vi "Capacitance PID-LS370.vi"() -> ()   [LabVIEW 2020]
doc: "This VI is meant to be used with the process control package (PID controller) and an MIO-series or Lab-PC data acquisition board. Connect the analog output to the analog input through the resistor-capacitor network shown on the front panel (scroll down to view it). The VI attempts to adjust the analog output so that the input (process variable or PV) equals the setpoint (SP). SP and PV are displayed on a strip chart. You can experiment with different controller tuning methods and try for the fastest settling time with the least overshoot.\n\nThe input span is -10 to +10 V, or 20V = 100%. The output span is 0 to +10 V, or 10V = 100%. PV and SP are in Volts. Your MIO board should be set up for differential input and -10 to +10 V range; the output should be unipolar, 10V (these are all factory defaults). If you elect to use other settings, run the configuration VIs as necessary.\n\nThe recommended network has a DC gain of 0.33, an effective deadtime of about 5 Sec., and an effective time constant of about 30 Sec."
uses:
  <vilib>/addons/control/pid/NI_PID__autopid compat.lvlib
panel:
  out "Trend 2":dbl(graph)
  in  "Heater Range":i32(ring)=4 items=["Off", "31.6 uA", "100 uA", "316 uA", "1.00 mA", "3.16 mA", "10.0 mA", "31.6 mA", "100 mA"]
  in  "Heater Resistance(½)":dbl=400.0
  in  "Lakeshore GPIB Address":refnum<visa-resource-name>="GPIB0::12::INSTR"
  out "Cycle #":i32
  in  "Bias":dbl format="%.2f"
  in  "gain scheduling":T1={"gain schedule"=[40.0, 70.0, 100.0], "PID parameters"=[{"Kc"=20.0, "Ti (min)"=0.008, "Td (min)"=0.006}, {"Kc"=20.0, "Ti (min)"=0.008, "Td (min)"=0.006}, {"Kc"=20.0, "Ti (min)"=0.008, "Td (min)"=0.006}], "scheduling input"=0} {"scheduling input" items=["Setpoint", "Process variable", "Controller output", "Gain scheduling input"]; "PID parameters"."Td (min)" format="%.4f"; "PID parameters"."Ti (min)" format="%.4f"; "PID parameters"."Kc" format="%#.3f"; "gain schedule" format="%.2f"}
  in  "?":bool
  in  "options":T2={"sp low"=-10.0, "sp high"=10.0, "out low"=0.0, "out high"=10.0, "hold (F)"=FALSE, "auto (T)"=TRUE, "pro. band (F)"=FALSE, "reverse acting (T)"=TRUE, "beta"=1.0, "linearity"=1.0, "dt (s)"=-1.0} {"dt (s)" format="%.2f"; "linearity" min=0.0 max=1.0 format="%.2f"; "sp low" format="%.2f"; "sp high" format="%.2f"; "out low" format="%.2e"; "out high" format="%.2e"; "beta" min=0.0 max=1.0 format="%.2f"}
  in  "STOP":bool
  in  "Setpoint (pF)":dbl(slide)=3300.0 min=3350.0 max=3380.0 step=0.0001 scale=3350.0..3380.0 scale format="%.2f"
  out "Output (W)":dbl(slide) scale=0.0..0.025 scale format="%#.2p"
  in  "Cycle Time (sec)":dbl=0.5 format="%.2f"
  in  "Manual Out (W)":dbl(knob) min=-4e-06 max=4e-06 scale=-100.0..100.0 scale format="%#.2p"
  out "Trend":cluster{"Setpoint (V)":dbl, "Setpoint (V)":dbl}(graph)
  # "SP & PV range:"
  # "Output range:"
  # "-1: default,using\nsystem clock"
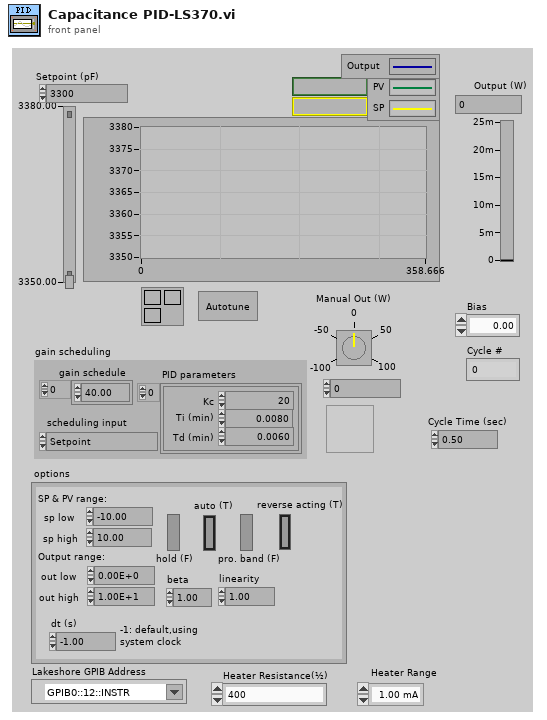
[diagram p1: front panel]
types:
  T1 = cluster{"gain schedule":dbl[], "PID parameters":cluster{"Kc":dbl, "Ti (min)":dbl, "Td (min)":dbl}[], "scheduling input":u16}
  T2 = cluster{"sp low":dbl, "sp high":dbl, "out low":dbl, "out high":dbl, "hold (F)":bool, "auto (T)":bool, "pro. band (F)":bool, "reverse acting (T)":bool, "beta":dbl, "linearity":dbl, "dt (s)":dbl}
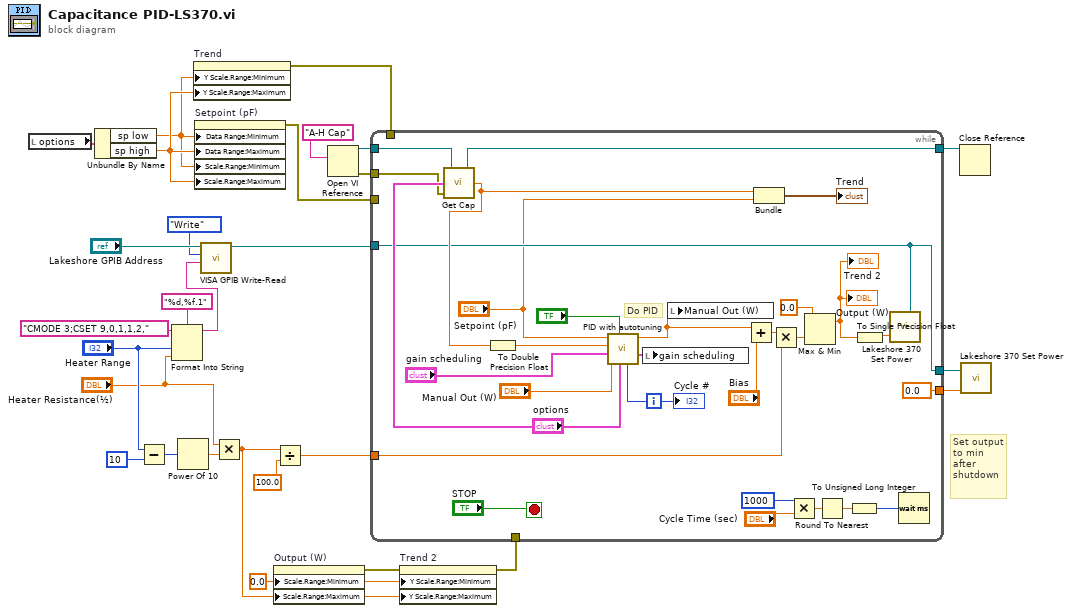
[diagram p0: block diagram]
diagram:
  w7 = 0.0 ("Scale.Range:Minimum")
  # "Set output \nto min after shutdown"
  n1 = local read "options"() -> (w11:T2)
  n2 = Unbundle By Name(w11) -> ("sp low"=w5:dbl, "sp high"=w6:dbl)
  n3 = Subtract(x="Heater Range", y=10) -> (x-y=w16:i32)
  n4 = Format Into String(format string="%d,%f.1" ("initial string"), initial string="CMODE 3;CSET 9,0,1,1,2,", "Heater Range", "Heater Resistance(½)") -> (resulting string=w18:string)  [unwired: 1 in, 1 out]
  n5 = Power Of 10(x=w16) -> (10^x=w13:dbl)
  n6 = property on="Trend" class="WFChart (strict)"("Y Scale.Range:Minimum"=w5, "Y Scale.Range:Maximum"=w6) -> (error out=w4:errorcluster)  [unwired: 2 in, 1 out]
  n7 = property on="Setpoint (pF)" class="Slide (strict)"("Data Range:Minimum"=w5, "Data Range:Maximum"=w6, "Scale.Range:Minimum"=w5, "Scale.Range:Maximum"=w6) -> (error out=w10:errorcluster)  [unwired: 2 in, 1 out]
  n8 = call "VISA GPIB Write-Read.vi"("Command"=w18, "Action"=enum16{"Write", "Read", "Write & Read"}."Write", "VISA resource name"="Lakeshore GPIB Address") -> ("dup VISA Session"=w21:refnum<visa-resource-name>)  [unwired: 5 in, 3 out]
  n9 = Multiply(x="Heater Resistance(½)", y=w13) -> (x*y=w3:dbl)
  n10 = property on="Output (W)" class="Slide (strict)"("Scale.Range:Minimum"=w7, "Scale.Range:Maximum"=w3) -> (error out=w9:errorcluster)  [unwired: 2 in, 1 out]
  n11 = Divide(x=w3, y=100.0) -> (x/y=w1:dbl)
  n12 = Open VI Reference(vi path="A-H Cap") -> (vi reference=w25:refnum<vi>, error out=w23:errorcluster)  [unwired: 5 in]
  n13 = property on="Trend 2" class="WFChart (strict)"(error in=w9, "Y Scale.Range:Minimum"=w7, "Y Scale.Range:Maximum"=w3) -> (error out=w8:errorcluster)  [unwired: 1 in, 1 out]
  n14 = while {
    tunnel: w23 -> [w43]
    tunnel: [w45] -> w24
    tunnel: w25 -> [w46]
    tunnel: [sgl 0.0] -> w27
    tunnel: [w36] -> w28
    tunnel: w21 -> [w36]
    tunnel: w10 -> [_]
    tunnel: w8 -> [_]
    tunnel: w4 -> [_]
    tunnel: w1 -> [w32]
    i -> [w51]
    stop <- "STOP" stop-if-true
    # "Do PID"
    n15 = call "Get Cap.vi"("error in"=w43, "options"="options", "VI Refnum 2"=w46) -> ("Setpoint (V)"=w42:dbl, "VI Refnum"=w45:refnum<vi>)  [unwired: 1 in]
    n16 = To Double Precision Float(number=w42) -> (double precision float=w47:dbl)
    n17 = call <vilib>:"PID with autotuning.vi"("iteration"=w51, "options"="options", "autotune? (F)"="?", "manual control"="Manual Out (W)", "gain scheduling"="gain scheduling", "process variable"=w47, "setpoint"="Setpoint (pF)") -> ("updated parameters"=w50:T1, "output"=w40:dbl)  [unwired: 2 in, 1 out]
    n18 = local write "gain scheduling"(w50) -> ()
    n19 = local write "Manual Out (W)"(w40) -> ()
    n20 = Add(x=w40, y="Bias") -> (x+y=w34:dbl)
    n21 = Bundle("Setpoint (V)"=w42, "Setpoint (pF)"="Setpoint (pF)") -> (→"Trend":cluster{"Setpoint (V)":dbl, "Setpoint (pF)":dbl})  [unwired: 1 in]
    n22 = Multiply(x=w34, y=w32) -> (x*y=w33:dbl)
    n23 = Multiply(x=1000, y="Cycle Time (sec)") -> (x*y=w54:dbl)
    n24 = Max & Min(x=0.0, y=w33) -> (max(x,y)=w30:dbl)  [unwired: 1 out]
    "Output (W)" <- w30
    "Trend 2" <- w30
    n25 = Round To Nearest(number=w54) -> (nearest integer value=w39:dbl)
    n26 = To Unsigned Long Integer(number=w39) -> (unsigned 32bit integer=w38:u32)
    n27 = To Single Precision Float(number=w30) -> (single precision float=w31:sgl)
    n28 = call "Lakeshore 370 Set Power.vi"("Heater Power (W)"=w31, "Lakeshore GPIB Address"=w36) -> ()
    n29 = Wait (ms)(milliseconds to wait=w38) -> ()  [unwired: 1 out]
    "Cycle #" <- w51
  }
  n30 = Close Reference(reference=w24) -> ()  [unwired: 1 in, 1 out]
  n31 = call "Lakeshore 370 Set Power.vi"("Heater Power (W)"=w27, "Lakeshore GPIB Address"=w28) -> ()
